vi "2D Zero Array.vi"(10 "Columns":i32, 11 "Rows":i32) -> (3 "Zero Array":dbl[][](array[numeric]))   [LabVIEW 2021]
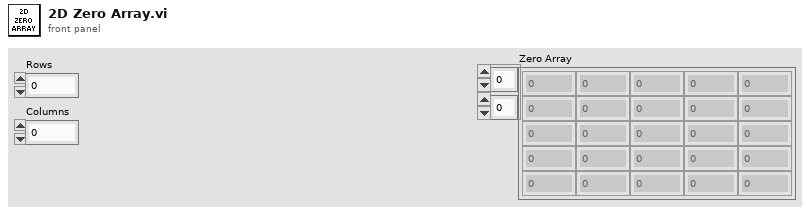
[diagram p1: front panel]
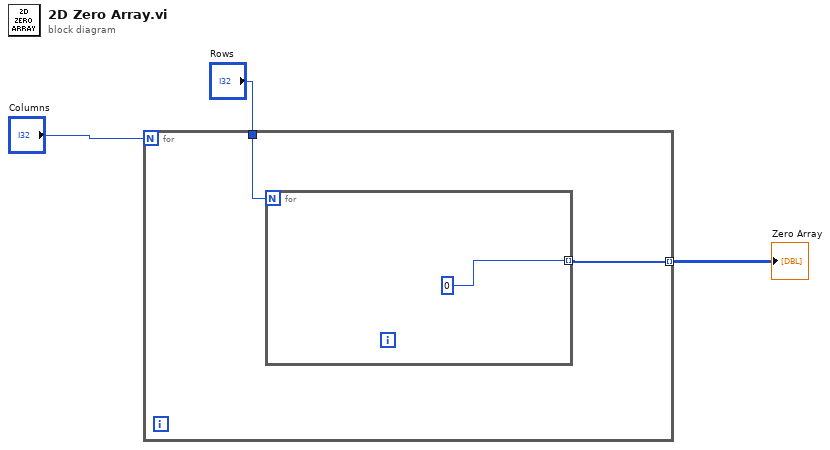
[diagram p0: block diagram]
diagram:
  n1 = for {
    N: "Columns" -> [_]
    tunnel: "Rows" -> [w5]
    tunnel: [w4] -> w1 mode=indexing
    n2 = for {
      N: w5 -> [_]
      tunnel: [0] -> w4 mode=indexing
    }
  }
  "Zero Array" <- w1
